vi "Begin.vi"   [LabVIEW 2019, in "LabPack.lvlib" / "Reader.lvclass"]
doc: "Starts the internal decoder. This is required to be called before any other decoding VIs are used. This creates a new buffer and tree, i.e. this will potentially allocate memory."
uses:
  Reader.lvclass
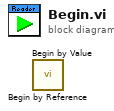
[diagram p0: block diagram]
diagram:
  n1 = call "Begin by Reference.vi"() -> ()  [unwired: 10 in, 2 out]
  n2 = call "Begin by Value.vi"() -> ()  [unwired: 10 in, 2 out]
